vi "UART_U8_Timeout.vi"(6 "断帧时间ms":u32=15, 8 "error in (no error)":errorcluster caption="错误输入（无错误）", 9 "超时s":dbl=0.1, 10 "写入字符串":string=">01 *idn?\n", 11 "BASE_COM":refnum<visa-resource-name>="COM1") -> (0 "error out":errorcluster caption="错误输出", 1 "OK":bool, 2 "读取字符串":string, 3 "BASE_COM_OUT":refnum<visa-resource-name>, 4 "使用时间ms":u32)   [LabVIEW 2015, in "UARTCOM.lvlib"]
uses:
  UARTCOM.lvlib
panel:
  # ">=10"
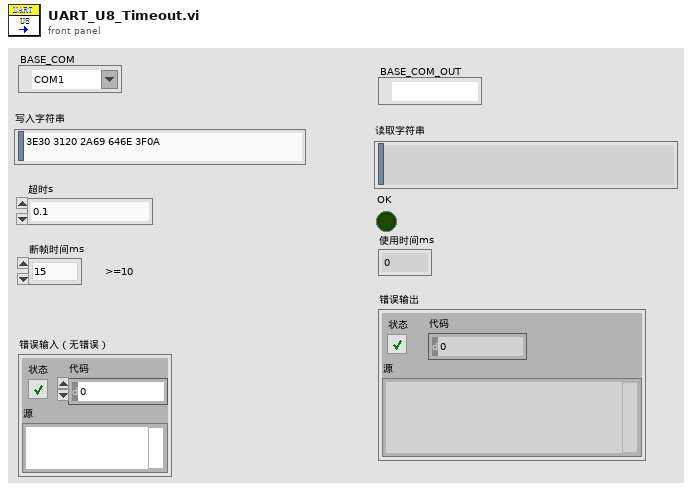
[diagram p1: front panel]
types:
  T1 = typedef "Semaphore RefNum" = refnum<k1>
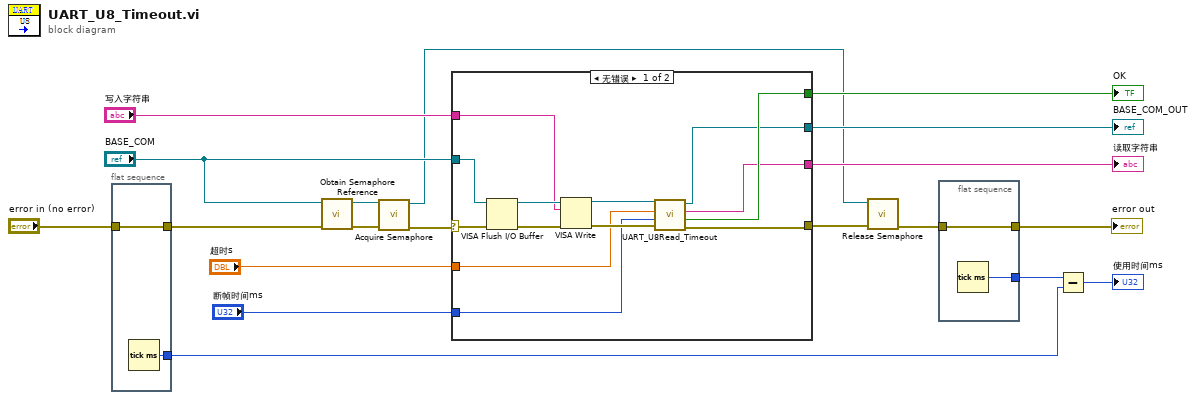
[diagram p0: block diagram]
diagram:
  n1 = flat-sequence {
    tunnel: "error in (no error)" -> [w21]
    tunnel: [w21] -> w6
    tunnel: [w20] -> w2
    frame #0 {
      n2 = Tick Count (ms)() -> (millisecond timer value=w20:u32)
    }
  }
  n3 = call <vilib>:"Obtain Semaphore Reference.vi"("error in (no error)"=w6, "name (unnamed)"="BASE_COM") -> ("error out"=w14:errorcluster, "semaphore"=w13:T1)  [unwired: 3 in, 1 out]
  n4 = call <vilib>:"Acquire Semaphore.vi"("error in (no error)"=w14, "semaphore"=w13) -> ("error out"=w11:errorcluster, "semaphore out"=w12:T1)  [unwired: 3 in, 1 out]
  n5 = case shown="无错误" w11 {
    selector: w11 -> [w34 w35]
    tunnel: "BASE_COM" -> [w32 w36]
    tunnel: [w25 w36] -> w19
    tunnel: "写入字符串" -> [w22 _]
    tunnel: [w26 _] -> w17
    tunnel: [w27 _] -> w16
    tunnel: [w24 w35] -> w10
    tunnel: "超时s" -> [w29 _]
    tunnel: "断帧时间ms" -> [w23 _]
    frame No Error {
      n6 = VISA Flush I/O Buffer(VISA resource name=w32, error in (no error)=w34) -> (VISA resource name out=w31:refnum<visa-resource-name>, error out=w33:errorcluster)  [unwired: 1 in]
      n7 = VISA Write(VISA resource name=w31, write buffer=w22, error in (no error)=w33) -> (VISA resource name out=w28:refnum<visa-resource-name>, error out=w30:errorcluster)  [unwired: 1 out]
      n8 = call "UART_U8Read_Timeout.vi"("error in (no error)"=w30, "断帧时间ms"=w23, "超时s"=w29, "BASE_COM"=w28) -> ("error out"=w24:errorcluster, "HasDat"=w27:bool, "Strout"=w26:string, "BASE_COM_OUT"=w25:refnum<visa-resource-name>)  [unwired: 4 in]
    }
    frame Error {
    }
  }
  "BASE_COM_OUT" <- w19
  "读取字符串" <- w17
  "OK" <- w16
  n9 = call <vilib>:"Release Semaphore.vi"("error in (no error)"=w10, "semaphore"=w12) -> ("error out"=w5:errorcluster)  [unwired: 4 in, 1 out]
  n10 = flat-sequence {
    tunnel: w5 -> [w38]
    tunnel: [w38] -> w4
    tunnel: [w37] -> w3
    frame #0 {
      n11 = Tick Count (ms)() -> (millisecond timer value=w37:u32)
    }
  }
  n12 = Subtract(x=w3, y=w2) -> (x-y=→"使用时间ms":u32)
  "error out" <- w4
